vi "Convert ASIIC to Hex String.vi"(4 "String":string) -> (1 "Hex String":string)   [LabVIEW 2020, in "CBOR.lvlib"]
doc: "Convert ASIIC string into Hexadecimal String."
uses:
  CBOR.lvlib
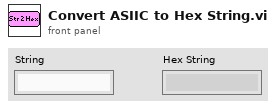
[diagram p1: front panel]
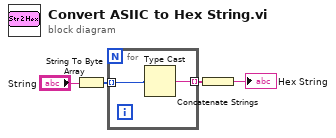
[diagram p0: block diagram]
diagram:
  n1 = String To Byte Array(string="String") -> (unsigned byte array=w3:u8[])
  n2 = for {
    tunnel: w3 -> [w6] mode=indexing
    tunnel: [w5] -> w1 mode=indexing
    n3 = Type Cast(x=w6) -> (*(type *) &x=w5:string)  [unwired: 1 in]
  }
  n4 = Concatenate Strings(w1) -> (→"Hex String":string)
